vi "SPD Data vs PM Level shift.vi"(8 "error in":errorcluster, 9 "Data shift":u8, 10 "PM Level in":u8[](array[numeric]), 11 "SPD Number in":u8[](array[numeric])) -> (0 "error out":errorcluster, 2 "PM Level out":u8[](array[numeric]), 3 "SPD Number out":u8[](array[numeric]))   [LabVIEW 2018]
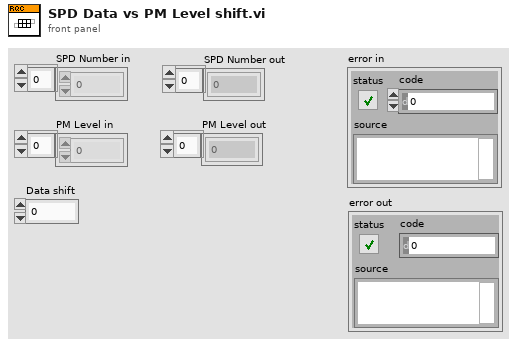
[diagram p1: front panel]
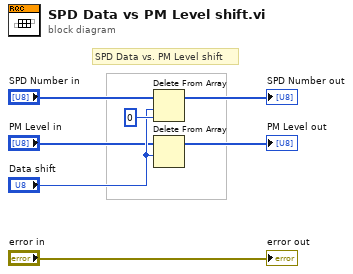
[diagram p0: block diagram]
diagram:
  # "SPD Data vs. PM Level shift"
  n1 = Delete From Array(array="SPD Number in", length="Data shift", index=0) -> (array with subset deleted=→"SPD Number out":u8[])  [unwired: 1 out]
  n2 = Delete From Array(array="PM Level in", length="Data shift") -> (array with subset deleted=→"PM Level out":u8[])  [unwired: 1 in, 1 out]
  "error out" <- "error in"
